vi "Wizard Strings.vi"() -> ()   [LabVIEW 2018]
panel:
  in  "Include Evaluation String Comment":string="IncludeEvalString"
  in  "Assert Conditional Disable Placement":string="CDS"
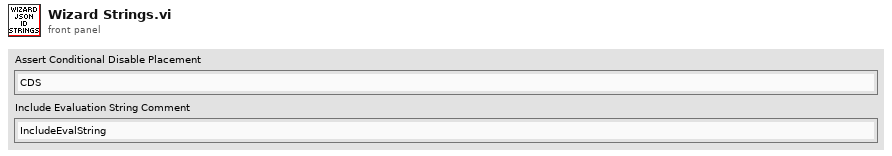
[diagram p1: front panel]
diagram:
